vi "Arduino.vi"() -> ()   [LabVIEW 2025]
uses:
  <vilib>/Instr/_visa.llb/VISA Configure Serial Port (Instr).vi
panel:
  out "Gauge":dbl(knob) scale=0.0..360.0
  out "Setpoint":dbl(knob) scale=0.0..360.0
  in  "OK Button":bool
  in  "Setpoint":string
  out "Posicion actual":i32
  out "Sensor":string
  in  "stop":bool
  in  "VISA resource name":refnum<visa-resource-name>
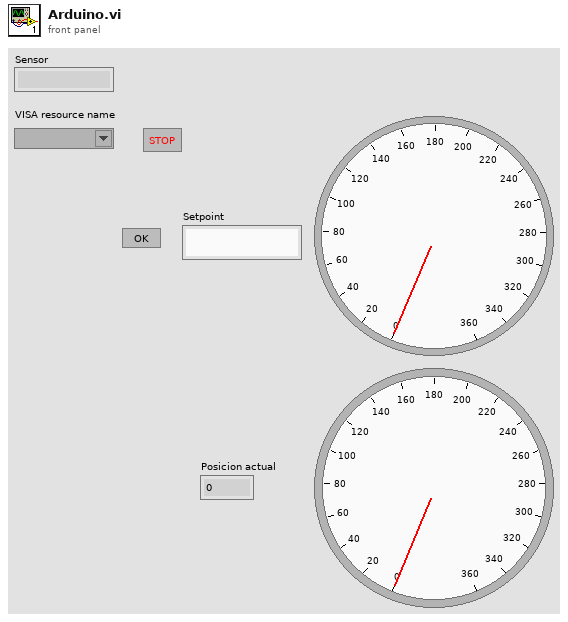
[diagram p1: front panel]
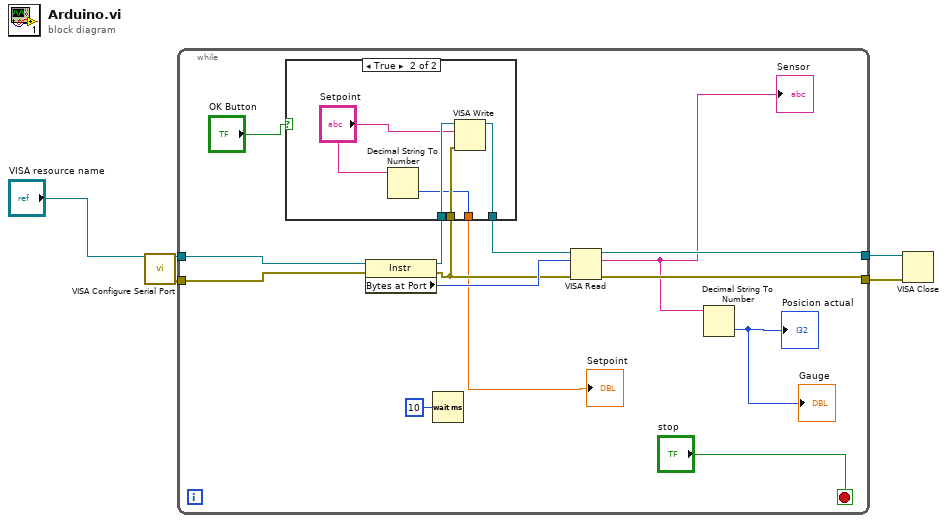
[diagram p0: block diagram]
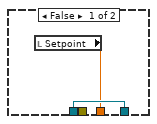
[diagram p2: hidden frame]
diagram:
  n1 = call-poly "VISA Configure Serial Port"("VISA resource name"="VISA resource name") -> ("VISA resource name out"=w4:refnum<visa-resource-name>, "error out"=w5:errorcluster)  [unwired: 13 in]
  n2 = while {
    tunnel: w5 -> [w18]
    tunnel: w4 -> [w12]
    tunnel: [w15] -> w3
    tunnel: [w16] -> w2
    stop <- "stop" stop-if-true
    n3 = property class="Instr"(reference=w12, error in=w18) -> (reference out=w10:refnum<visa-resource-name>, error out=w11:errorcluster, "Bytes at Port"=w17:u32)
    n4 = case shown="True" "OK Button" {
      tunnel: w11 -> [_ w26]
      tunnel: w10 -> [w21 w25]
      tunnel: [w21 w24] -> w9
      tunnel: [w20 w22] -> w7
      frame False {
        n5 = local read "Setpoint"() -> (w20:dbl)
      }
      frame True {
        n6 = Decimal String To Number(string="Setpoint") -> (number=w22:i32)  [unwired: 2 in, 1 out]
        n7 = VISA Write(VISA resource name=w25, write buffer="Setpoint", error in (no error)=w26) -> (VISA resource name out=w24:refnum<visa-resource-name>)  [unwired: 2 out]
      }
    }
    "Setpoint" <- w7
    n8 = Wait (ms)(milliseconds to wait=u32 10) -> ()  [unwired: 1 out]
    n9 = VISA Read(VISA resource name=w9, byte count=w17, error in (no error)=w11) -> (VISA resource name out=w15:refnum<visa-resource-name>, read buffer=w14:string, error out=w16:errorcluster)  [unwired: 1 out]
    "Sensor" <- w14
    n10 = Decimal String To Number(string=w14) -> (number=→"Posicion actual" →"Gauge":i32)  [unwired: 2 in, 1 out]
  }
  n11 = VISA Close(VISA resource name=w3, error in (no error)=w2) -> ()  [unwired: 1 out]
